vi "Configure Scan.vi"(8 "error in (no error)":errorcluster, 9 "Sample Count (1)":i32=6, 10 "Channel List (101:110)":string="110,113:115,119:120", 11 "DMM":refnum<visa-resource-name>="COM1") -> (0 "error out":errorcluster, 3 "VISA resource name out":refnum<visa-resource-name>)   [LabVIEW 2015]
uses:
  <instrlib>/Keithley 27XX/Keithley 27XX.lvlib
panel:
  out "error out 2":errorcluster
  in  "Serial Configuration":T1={"Baud Rate (19200)"=19200, "Flow Control (1: XON/XOFF)"=1, "Termination Char (0:CR)"=0} {"Termination Char (0:CR)" items=["CR", "LF"]; "Flow Control (1: XON/XOFF)" items=["None", "XON/XOFF", "RTS/CTS (2701 Only)", "XON/XOFF & RTS/CTS (2701 Only)"]; "Baud Rate (19200)" items=["300"=300, "600"=600, "1200"=1200, "2400"=2400, "4800"=4800, "9600"=9600, "19.2k"=19200, "38.4k (2701 Only)"=38400, "57.6k (2701 Only)"=57600, "115.2k (2701 Only)"=115200]}
  in  "Timeout (5000 milliseconds)":u32=5000
  in  "Function (0: DC Voltage)":u16(ring) items=["DC Voltage", "AC Voltage", "DC Current", "AC Current", "Resistance", "Four-Wire Resistance", "Temperature (C)", "Frequency", "Period", "Continuity"]
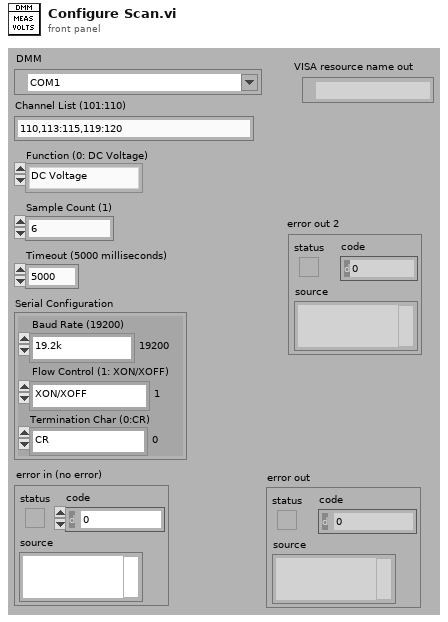
[diagram p1: front panel]
types:
  T1 = cluster{"Baud Rate (19200)":u32, "Flow Control (1: XON/XOFF)":u16, "Termination Char (0:CR)":u16}
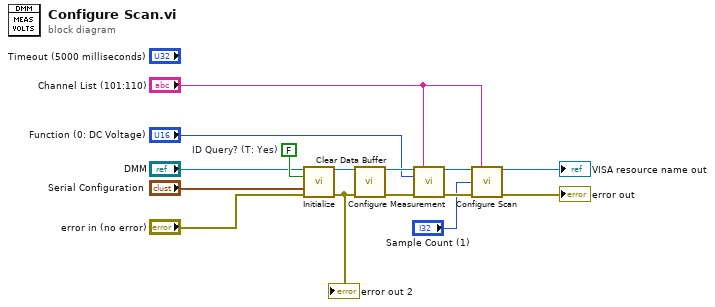
[diagram p0: block diagram]
diagram:
  w4 = FALSE  # ID Query? (T: Yes)
  n1 = call <instrlib>:"Initialize.vi"("VISA resource name"="DMM", "ID Query? (T: Yes)"=w4, "Serial Configuration"="Serial Configuration", "error in (no error)"="error in (no error)") -> ("VISA resource name out"=w10:refnum<visa-resource-name>, "error out"=w11:errorcluster)  [unwired: 10 in]
  "error out 2" <- w11
  n2 = call <instrlib>:"Clear Data Buffer.vi"("VISA resource name"=w10, "error in (no error)"=w11) -> ("VISA resource name out"=w13:refnum<visa-resource-name>, "error out"=w12:errorcluster)  [unwired: 12 in]
  n3 = call <instrlib>:"Configure Measurement.vi"("VISA resource name"=w13, "Scan List (Empty)"="Channel List (101:110)", "Function (0: DC Voltage)"="Function (0: DC Voltage)", "error in (no error)"=w12) -> ("VISA resource name out"=w15:refnum<visa-resource-name>, "error out"=w14:errorcluster)  [unwired: 10 in]
  n4 = call <instrlib>:"Configure Scan.vi"("VISA resource name"=w15, "Channel List (101:110)"="Channel List (101:110)", "Sample Count (100)"="Sample Count (1)", "error in (no error)"=w14) -> ("VISA resource name out"=→"VISA resource name out":refnum<visa-resource-name>, "error out"=→"error out":errorcluster)  [unwired: 10 in]
